vi "Stim ASICs Registers and RAMs.vi"() -> (0 "RAM 2":i32[](array[numeric]), 1 "RAM1":i32[](array[numeric]), 2 "Stim ASIC's Register":u32[](array[numeric]), 3 "Stim ASIC's":string[][](array[string]))   [LabVIEW 2010]
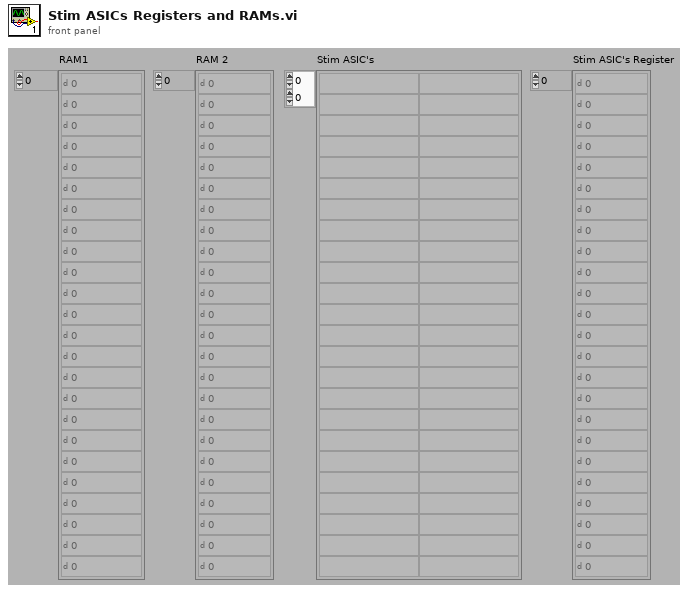
[diagram p1: front panel]
types:
  T1 = enum32{"invalid app kind", "Development System", "Run Time System", "Student Edition", "Embedded LabVIEW", "Evaluation", "Custom"}
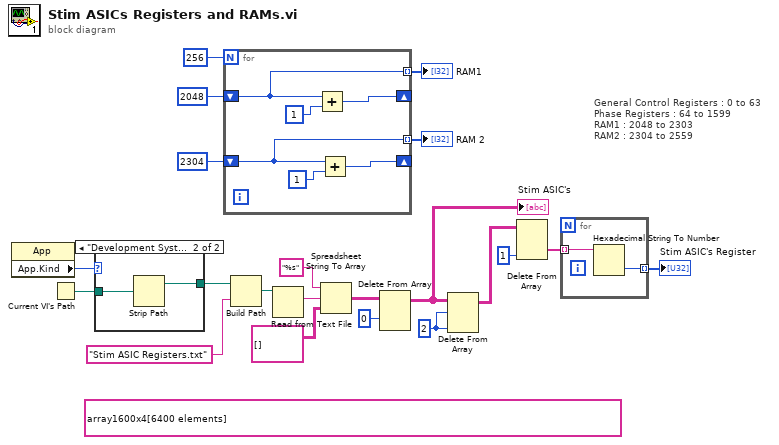
[diagram p0: block diagram]
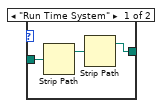
[diagram p2: hidden frame]
diagram:
  (unwired) string[][] array1600x4[6400 elements] ("Stim ASIC's")
  w5 = 2 ("disabled index (col)")
  # "General Control Registers : 0 to 63\nPhase Registers : 64 to 1599\nRAM1 : 2048 to 2303\nRAM2 : 2304 to 2559"
  n1 = property class="App"() -> ("App.Kind"=w3:T1)  [unwired: 2 in, 2 out]
  n2 = Current VI's Path() -> (path=w14:path)
  n3 = case shown="\"Development System\", Default" w3 {
    tunnel: w14 -> [w24 w26]
    tunnel: [w22 w25] -> w12
    frame "Run Time System" {
      n4 = Strip Path(path=w24) -> (stripped path=w23:path)  [unwired: 1 out]
      n5 = Strip Path(path=w23) -> (stripped path=w22:path)  [unwired: 1 out]
    }
    frame "Development System", Default {
      n6 = Strip Path(path=w26) -> (stripped path=w25:path)  [unwired: 1 out]
    }
  }
  n7 = for {
    N: 256 -> [_]
    shift-right: [w31] -> _
    shift-left: 2048 -> [w30]
    tunnel: [w30] -> w18 mode=indexing
    shift-right: [w29] -> _
    shift-left: 2304 -> [w27]
    tunnel: [w27] -> w17 mode=indexing
    n8 = Add(x=w30, y=1) -> (x+y=w31:i32)
    n9 = Add(x=w27, y=1) -> (x+y=w29:i32)
  }
  "RAM1" <- w18
  "RAM 2" <- w17
  n10 = Build Path(base path=w12, name or relative path="Stim ASIC Registers.txt") -> (appended path=w8:path)
  n11 = Read from Text File(file (use dialog)=w8) -> (text=w11:string)  [unwired: 3 in, 3 out]
  n12 = Spreadsheet String To Array(format string="%s", spreadsheet string=w11, array type (2D Dbl)=string[][] []) -> (array=w7:string[][])  [unwired: 1 in]
  n13 = Delete From Array(array=w7, index (row)=0 ("disabled index (col)")) -> (array with subset deleted=w1:string[][])  [unwired: 2 in, 1 out]
  "Stim ASIC's" <- w1
  n14 = Delete From Array(array=w1, length=w5, index (col)=w5) -> (array with subset deleted=w2:string[][])  [unwired: 1 in, 1 out]
  n15 = Delete From Array(array=w2, index (col)=1 ("disabled index (col)")) -> (deleted portion=w15:string[])  [unwired: 2 in, 1 out]
  n16 = for {
    tunnel: w15 -> [w34] mode=indexing
    tunnel: [w33] -> w4 mode=indexing
    n17 = Hexadecimal String To Number(string=w34) -> (number=w33:u32)  [unwired: 2 in, 1 out]
  }
  "Stim ASIC's Register" <- w4
